vi "DrawArrow.vi"(9 "angle (deg)":dbl, 10 "velocity":cluster{dbl, dbl}, 11 "end of line":cluster{dbl, dbl}) -> (3 "arrow":cluster{dbl, dbl}[](array[cluster]))   [LabVIEW 2025]
panel:
  out "new picture":picture
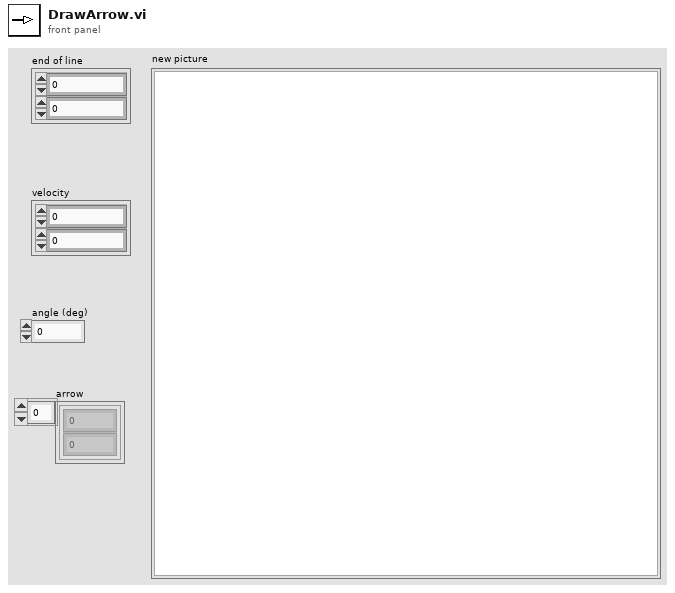
[diagram p1: front panel]
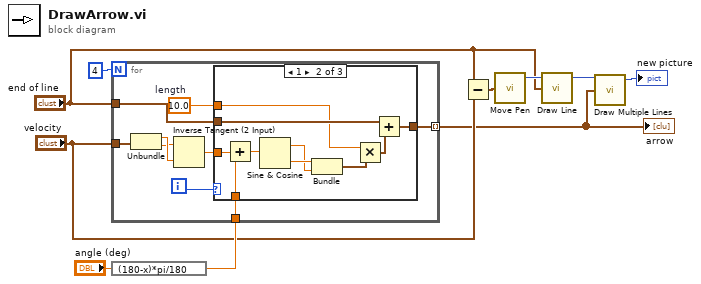
[diagram p0: block diagram]
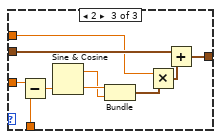
[diagram p3: hidden frame]
diagram:
  n1 = expression code="(180-x)*pi/180"("angle (deg)") -> (w10:dbl)
  n2 = for {
    N: 4 -> [_]
    tunnel: [w18] -> w1 mode=indexing
    tunnel: "velocity" -> [w15]
    tunnel: w10 -> [w14]
    tunnel: "end of line" -> [w11]
    i -> [w19]
    w13 = 10.0  # length
    n3 = Unbundle(w15) -> (w17:dbl, w16:dbl)
    n4 = Inverse Tangent (2 Input)(1:w17, 2:w16) -> (0:w12:dbl)
    n5 = case shown="1" w19 {
      tunnel: [w20 w22 w32] -> w18
      tunnel: w11 -> [w20 w24 w34]
      tunnel: w12 -> [_ w26 w36]
      tunnel: w14 -> [_ w25 w35]
      tunnel: w13 -> [_ w21 w31]
      frame 0, Default {
      }
      frame 1 {
        n6 = Add(x=w26, y=w25) -> (x+y=w30:dbl)
        n7 = Sine & Cosine(0:w30) -> (1:w28:dbl, 2:w29:dbl)
        n8 = Bundle(w29, w28) -> (w27:cluster{dbl, dbl})  [unwired: 1 in]
        n9 = Multiply(x=w21, y=w27) -> (x*y=w23:cluster{dbl, dbl})
        n10 = Add(x=w24, y=w23) -> (x+y=w22:cluster{dbl, dbl})
      }
      frame 2 {
        n11 = Subtract(x=w36, y=w35) -> (x-y=w40:dbl)
        n12 = Sine & Cosine(0:w40) -> (1:w38:dbl, 2:w39:dbl)
        n13 = Bundle(w39, w38) -> (w37:cluster{dbl, dbl})  [unwired: 1 in]
        n14 = Multiply(x=w31, y=w37) -> (x*y=w33:cluster{dbl, dbl})
        n15 = Add(x=w34, y=w33) -> (x+y=w32:cluster{dbl, dbl})
      }
    }
  }
  "arrow" <- w1
  n16 = Subtract(x="end of line", y="velocity") -> (x-y=w4:cluster{dbl, dbl})
  n17 = call <vilib>:"Move Pen.vi"("new position"=w4) -> ("new picture"=w6:picture)  [unwired: 4 in]
  n18 = call <vilib>:"Draw Line.vi"("picture"=w6, "end point"="end of line") -> ("new picture"=w5:picture)  [unwired: 7 in]
  n19 = call <vilib>:"Draw Multiple Lines.vi"("picture"=w5, "line endpoints"=w1) -> ("new picture"=→"new picture":picture)  [unwired: 7 in]
